vi "FTW-Request-Unknown.vi"(0 "FTW Incoming Request":refnum<class "FTW-Request.lvclass">, 11 "error in":errorcluster) -> (4 "FTW Incoming Request out":refnum<class "FTW-Request.lvclass">, 15 "error out":errorcluster)   [LabVIEW 2013, in "FTW-Actor.lvlib" / "FTW-Request.lvclass"]
uses:
  FTW-Request.lvclass
  FTW-Request.lvclass/FTW-Request.ctl
panel:
  # "Inputs"
  # "Outputs"
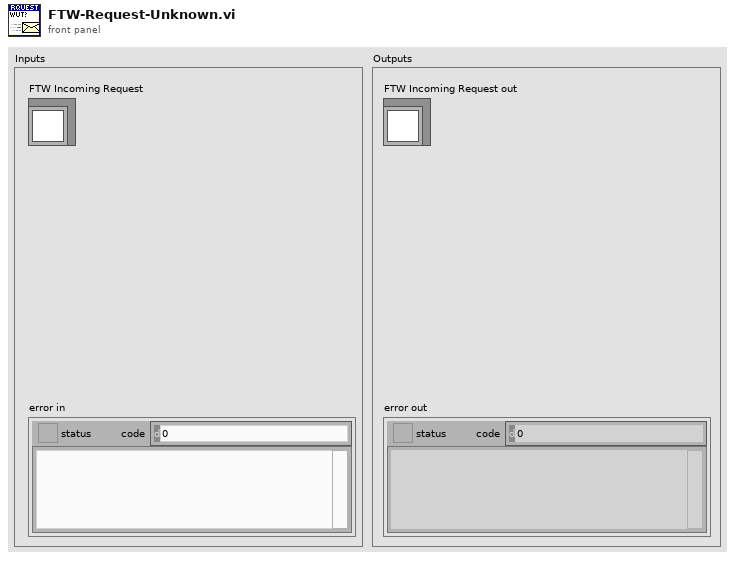
[diagram p1: front panel]
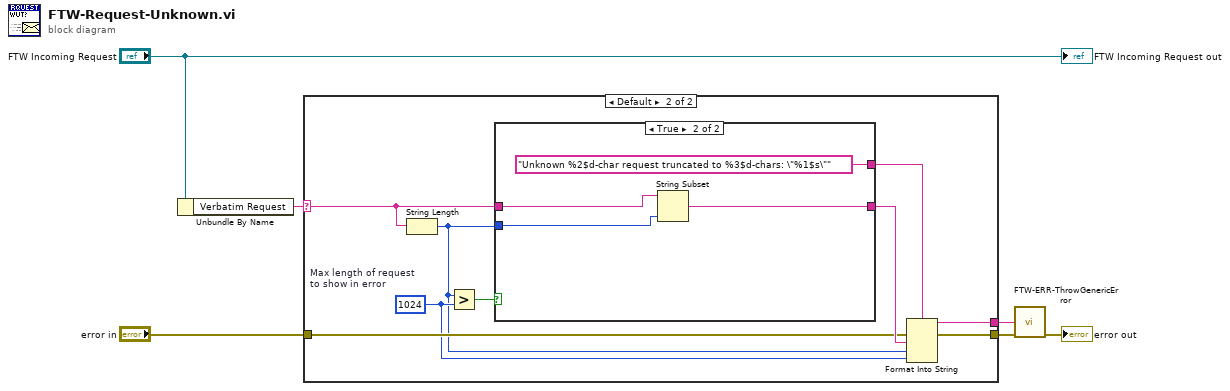
[diagram p0: block diagram]
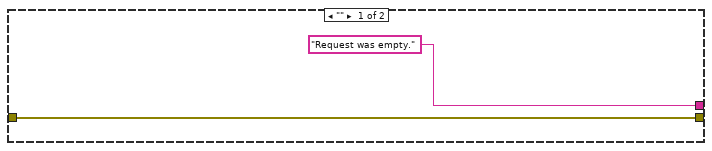
[diagram p2: hidden frame]
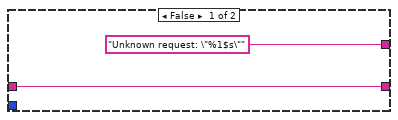
[diagram p3: hidden frame]
diagram:
  n1 = Unbundle By Name("FTW Incoming Request") -> ("Verbatim Request"=w4:string)
  n2 = case shown="Default" w4 {
    selector: w4 -> [_ w11]
    tunnel: [w7 w10] -> w3
    tunnel: "error in" -> [w7 w14]
    tunnel: ["Request was empty." ("Error Message") w9] -> w1
    frame "" {
    }
    frame Default {
      w13 = 1024  # Max length of request to show in error
      n3 = String Length(string=w11) -> (length=w12:i32)
      n4 = Greater?(x=w12, y=w13) -> (0:w17:bool)
      n5 = case shown="True" w17 {
        tunnel: w11 -> [w19 w23]
        tunnel: [w19 w21] -> w16
        tunnel: ["Unknown request: \"%1$s\"" ("format string") "Unknown %2$d-char request truncated to %3$d-chars: \"%1$s\"" ("format string")] -> w15
        tunnel: w12 -> [_ w22]
        frame False {
        }
        frame True {
          n6 = String Subset(string=w23, length (rest)=w22) -> (substring=w21:string)  [unwired: 1 in]
        }
      }
      n7 = Format Into String(format string=w15, error in=w14, w16, w12, w13) -> (resulting string=w9:string, error out=w10:errorcluster)  [unwired: 1 in]
    }
  }
  n8 = call "FTW-ERR-ThrowGenericError.vi"("Error Message"=w1, "error in"=w3) -> ("error out"=→"error out":errorcluster)  [unwired: 13 in]
  "FTW Incoming Request out" <- "FTW Incoming Request"
